vi "保持时间脚本.vi"(8 "4-wire":bool, 9 "强制时序":bool, 11 "维持时间":T1 {"ΔT" format="%#_6ps"; "T" format="%#_6ps"; "NPLC" min=0.001 max=25.0 step=0.001; "+ limit I" min=1e-08 max=3.0 format="%#_6pA"; "+ V" min=-40.0 max=40.0 format="%#_6pV"}) -> (3 "Script":string)   [LabVIEW 2020, in "功能选择.xctl"]
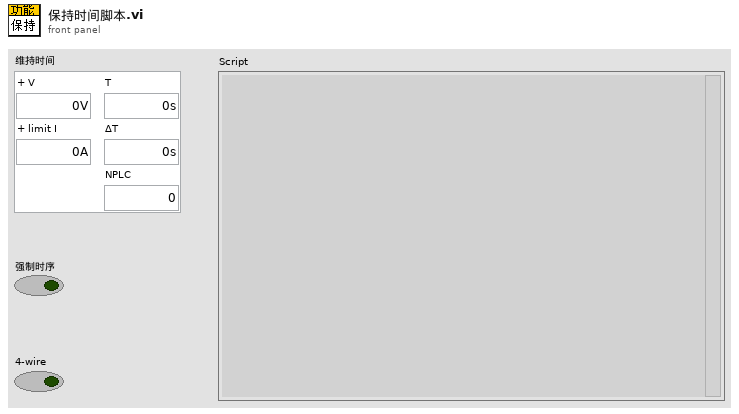
[diagram p1: front panel]
types:
  T1 = typedef "功能选择.xctl/保持时间.ctl" = cluster{"+ V":dbl, "+ limit I":dbl, "T":dbl, "ΔT":dbl, "NPLC":dbl}
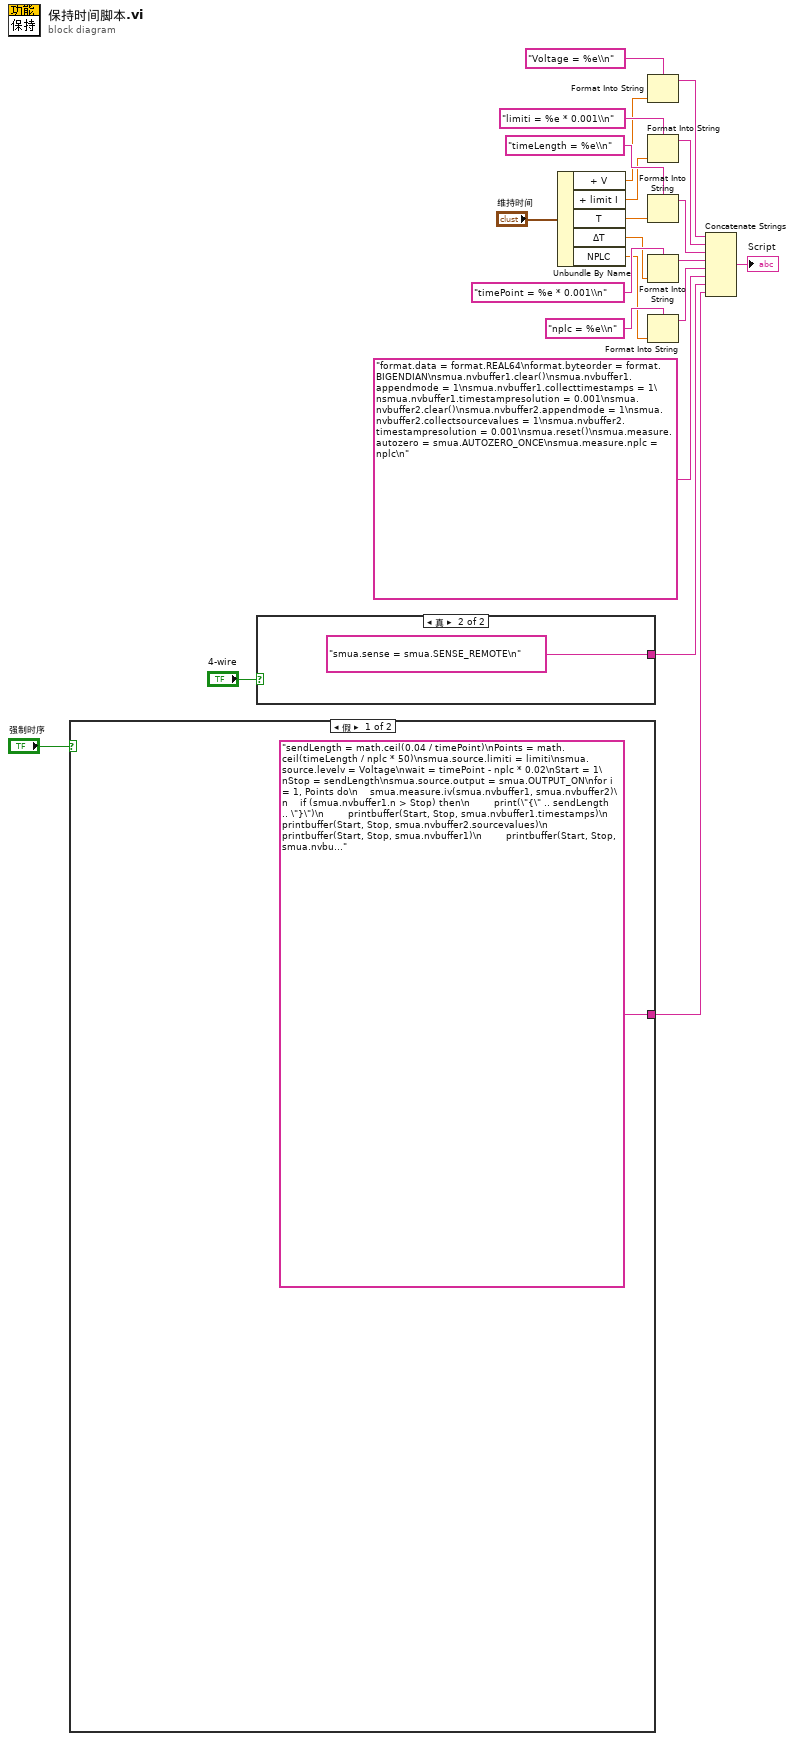
[diagram p0: block diagram]
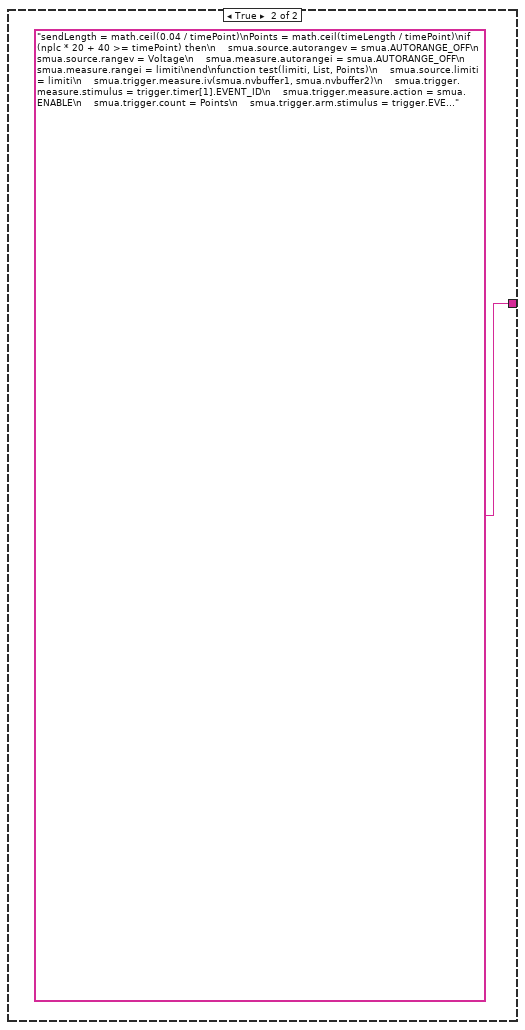
[diagram p2: hidden frame]
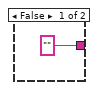
[diagram p3: hidden frame]
diagram:
  n1 = case shown="假" "强制时序" {
    tunnel: ["sendLength = math.ceil(0.04 / timePoint)\nPoints = math.ceil(timeLength / nplc * 50)\nsmua.source.limiti = limiti\nsmua.source.levelv = Voltage\nwait = timePoint - nplc * 0.02\nStart = 1\nStop = sendLength\nsmua.source.output = smua.OUTPUT_ON\nfor i = 1, Points do\n    smua.measure.iv(smua.nvbuffer1, smua.nvbuffer2)\n    if (smua.nvbuffer1.n > Stop) then\n        print(\"{\" .. sendLength .. \"}\")\n        printbuffer(Start, Stop, smua.nvbuffer1.timestamps)\n        printbuffer(Start, Stop, smua.nvbuffer2.sourcevalues)\n        printbuffer(Start, Stop, smua.nvbuffer1)\n        printbuffer(Start, Stop, smua.nvbuffer2)\n        Start = Start + sendLength\n        Stop = Stop + sendLength\n    end\n    if (wait * 1000 > 1) then\n        delay(wait)\n    end\nend\nsmua.source.output = smua.OUTPUT_OFF\nStop = Points\nprint(\"{\" .. Stop - Start + 1 .. \"}\")\nprintbuffer(Start, Stop, smua.nvbuffer1.timestamps)\nprintbuffer(Start, Stop, smua.nvbuffer2.sourcevalues)\nprintbuffer(Start, Stop, smua.nvbuffer1)\nprintbuffer(Start, Stop, smua.nvbuffer2)\nprint(\"{done}\")\nreset()" "sendLength = math.ceil(0.04 / timePoint)\nPoints = math.ceil(timeLength / timePoint)\nif (nplc * 20 + 40 >= timePoint) then\n    smua.source.autorangev = smua.AUTORANGE_OFF\n    smua.source.rangev = Voltage\n    smua.measure.autorangei = smua.AUTORANGE_OFF\n    smua.measure.rangei = limiti\nend\nfunction test(limiti, List, Points)\n    smua.source.limiti = limiti\n    smua.trigger.measure.iv(smua.nvbuffer1, smua.nvbuffer2)\n    smua.trigger.measure.stimulus = trigger.timer[1].EVENT_ID\n    smua.trigger.measure.action = smua.ENABLE\n    smua.trigger.count = Points\n    smua.trigger.arm.stimulus = trigger.EVENT_ID\n    trigger.timer[1].reset()\n    trigger.timer[1].stimulus = smua.trigger.ARMED_EVENT_ID\n    trigger.timer[1].passthrough = false\n    trigger.timer[1].delay = timePoint\n    trigger.timer[1].count = Points\n    smua.trigger.initiate()\n    smua.trigger.arm.set()\nend\nfunction sendData()\n    repeat\n        if (bit.test(status.operation.instrument.smua.condition, 4) == false) then\n            return\n        elseif (smua.nvbuffer1.n > Stop) then\n            print(\"{\" .. sendLength .. \"}\")\n            printbuffer(Start, Stop, smua.nvbuffer1.timestamps)\n            printbuffer(Start, Stop, smua.nvbuffer2.sourcevalues)\n            printbuffer(Start, Stop, smua.nvbuffer1)\n            printbuffer(Start, Stop, smua.nvbuffer2)\n            Start = Start + sendLength\n            Stop = Stop + sendLength\n        end\n        delay(timePoint)\n    until (false)\nend\nfunction sendLastData()\n    Stop = smua.nvbuffer1.n\n    print(\"{\" .. Stop - Start + 1 .. \"}\")\n    printbuffer(Start, Stop, smua.nvbuffer1.timestamps)\n    printbuffer(Start, Stop, smua.nvbuffer2.sourcevalues)\n    printbuffer(Start, Stop, smua.nvbuffer1)\n    printbuffer(Start, Stop, smua.nvbuffer2)\n    print(\"{done}\")\nend\nStart = 1\nStop = sendLength\nsmua.source.levelv = Voltage\nsmua.source.output = smua.OUTPUT_ON\ntest(limiti, List, Points)\nsendData()\nsmua.source.output = smua.OUTPUT_OFF\nsendLastData()\nreset()"] -> w12
    frame False {
    }
    frame True {
    }
  }
  n2 = case shown="真" "4-wire" {
    tunnel: ["" "smua.sense = smua.SENSE_REMOTE\n"] -> w11
    frame False {
    }
    frame True {
    }
  }
  n3 = Unbundle By Name("维持时间") -> ("+ V"=w6:dbl, "+ limit I"=w5:dbl, "T"=w4:dbl, "ΔT"=w3:dbl, "NPLC"=w2:dbl)
  n4 = Format Into String(format string="Voltage = %e\\n" ("格式字符串"), w6) -> (resulting string=w20:string)  [unwired: 2 in, 1 out]
  n5 = Format Into String(format string="limiti = %e * 0.001\\n" ("格式字符串"), w5) -> (resulting string=w15:string)  [unwired: 2 in, 1 out]
  n6 = Format Into String(format string="timeLength = %e\\n", w4) -> (resulting string=w14:string)  [unwired: 2 in, 1 out]
  n7 = Format Into String(format string="timePoint = %e * 0.001\\n" ("格式字符串"), w3) -> (resulting string=w9:string)  [unwired: 2 in, 1 out]
  n8 = Format Into String(format string="nplc = %e\\n", w2) -> (resulting string=w8:string)  [unwired: 2 in, 1 out]
  n9 = Concatenate Strings(w20, w15, w14, w9, w8, "format.data = format.REAL64\nformat.byteorder = format.BIGENDIAN\nsmua.nvbuffer1.clear()\nsmua.nvbuffer1.appendmode = 1\nsmua.nvbuffer1.collecttimestamps = 1\nsmua.nvbuffer1.timestampresolution = 0.001\nsmua.nvbuffer2.clear()\nsmua.nvbuffer2.appendmode = 1\nsmua.nvbuffer2.collectsourcevalues = 1\nsmua.nvbuffer2.timestampresolution = 0.001\nsmua.reset()\nsmua.measure.autozero = smua.AUTOZERO_ONCE\nsmua.measure.nplc = nplc\n", w11, w12) -> (→"Script":string)
